vi "Test read multiple pulses.vi"() -> ()   [LabVIEW 2023]
uses:
  <vilib>/DAQmx/create/channels.llb/DAQmx Create Channel (CI-Count Edges).vi
  <vilib>/DAQmx/configure/timing.llb/DAQmx Timing (Sample Clock).vi
  <vilib>/DAQmx/create/channels.llb/DAQmx Create Channel (CO-Pulse Generation-Frequency).vi
  <vilib>/DAQmx/configure/timing.llb/DAQmx Timing (Implicit).vi
  <vilib>/DAQmx/miscellaneous.llb/DAQmx Fill In Error Info.vi
  <vilib>/DAQmx/read.llb/DAQmx Read (Counter 1D U32 1Chan NSamp).vi
  <resource>/objmgr/daqmx.rc
panel:
  out "error out":errorcluster
  in  "# of pulses in train":i32=1000
  out "Actual Duty Cycle":dbl
  out "Actual Frequency":dbl
  in  "Duty Cycle":dbl=0.5 format="%.6f"
  in  "Frequency":dbl=1.0 format="%.6f"
  in  "Output Terminal":tag="/Dev1/PFI12"
  in  "Counter 2":tag="Dev1/ctr0"
  in  "Active Edge":i32(ring)=10280 items=["Rising"=10280, "Falling"=10171]
  in  "Input Terminal":tag="PFI8"
  in  "Counter":tag="Dev1/ctr0"
  in  "Sample Rate":dbl=1000.0
  in  "Sample Clock Source":tag="PFI0"
  in  "Samples per Loop":i32=100
  in  "Stop":bool
  out "Data":u32[](array[numeric])
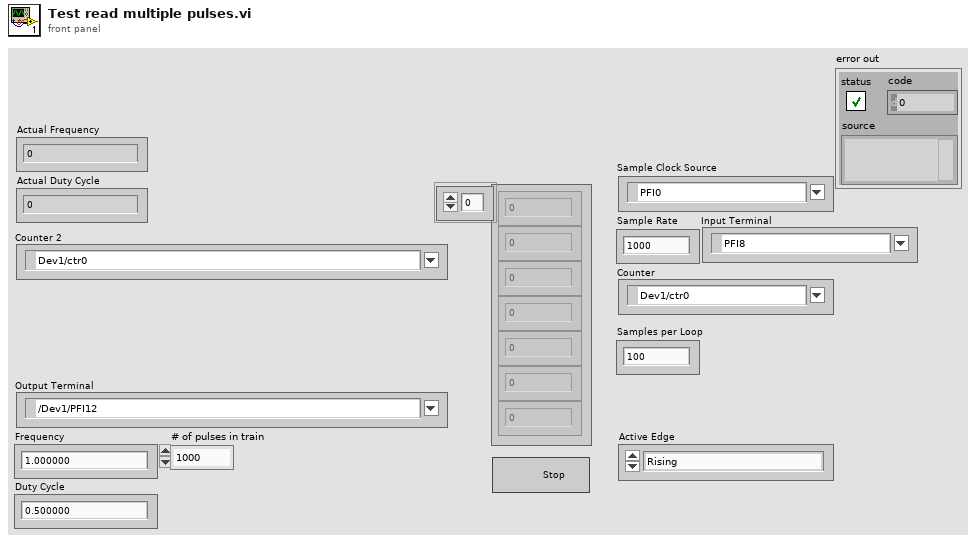
[diagram p1: front panel]
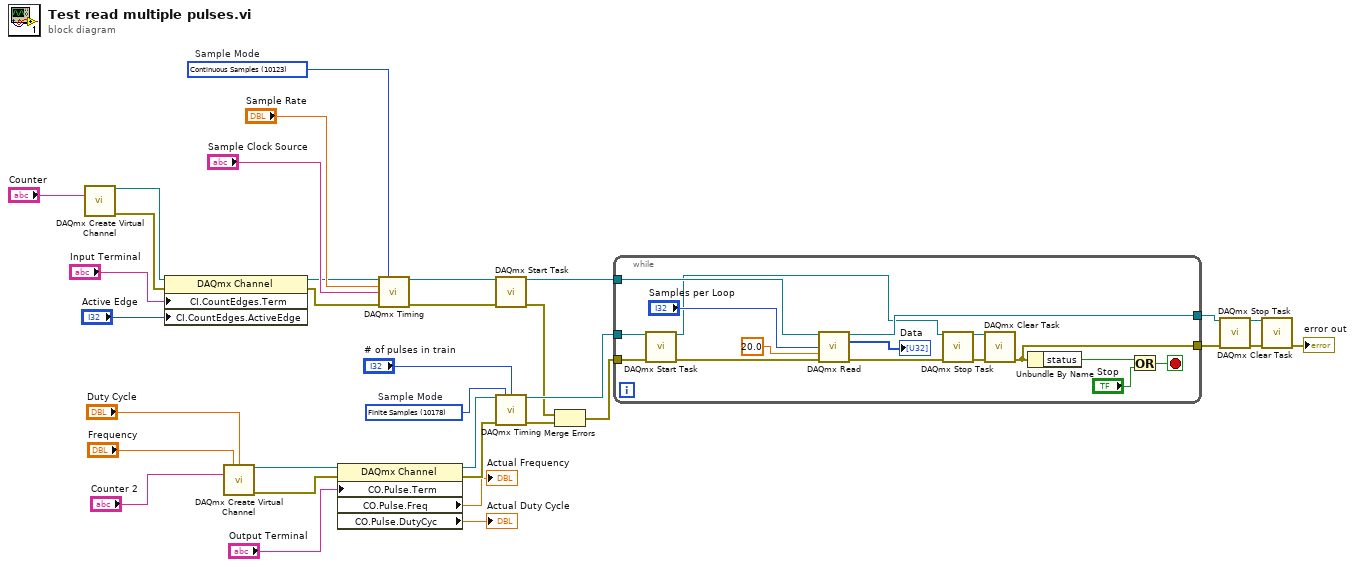
[diagram p0: block diagram]
diagram:
  w17 = 10178 items=["Finite Samples"=10178, "Continuous Samples"=10123, "Hardware Timed Single Point"=12522]  # Sample Mode
  w32 = 10123 items=["Finite Samples"=10178, "Continuous Samples"=10123, "Hardware Timed Single Point"=12522]  # Sample Mode
  n1 = call-poly <vilib>:"DAQmx Create Virtual Channel.vi"("counter"="Counter") -> ("task out"=w27:refnum<k21>, "error out"=w24:errorcluster)  [unwired: 13 in]
  n2 = property class="DAQmx Channel"(reference=w27, error in=w24, "CI.CountEdges.Term"="Input Terminal", "CI.CountEdges.ActiveEdge"="Active Edge") -> (reference out=w26:refnum<k21>, error out=w25:errorcluster)
  n3 = call-poly <vilib>:"DAQmx Create Virtual Channel.vi"("frequency"="Frequency", "duty cycle"="Duty Cycle", "counter"="Counter 2") -> ("task out"=w13:refnum<k21>, "error out"=w12:errorcluster)  [unwired: 11 in]
  n4 = property class="DAQmx Channel"(reference=w13, error in=w12, "CO.Pulse.Term"="Output Terminal") -> (reference out=w9:refnum<k21>, error out=w10:errorcluster, "CO.Pulse.Freq"=→"Actual Frequency":dbl, "CO.Pulse.DutyCyc"=→"Actual Duty Cycle":dbl)
  n5 = call-poly <vilib>:"DAQmx Timing.vi"("task/channels in"=w26, "sample mode"=w32, "rate"="Sample Rate", "source"="Sample Clock Source", "error in"=w25) -> ("task out"=w23:refnum<k21>, "error out"=w22:errorcluster)  [unwired: 9 in]
  n6 = call <vilib>:"DAQmx Start Task.vi"("task/channels in"=w23, "error in"=w22) -> ("task out"=w31:refnum<k21>, "error out"=w2:errorcluster)  [unwired: 12 in]
  n7 = call-poly <vilib>:"DAQmx Timing.vi"("task/channels in"=w9, "sample mode"=w17, "samples per channel"="# of pulses in train", "error in"=w10) -> ("task out"=w15:refnum<k21>, "error out"=w14:errorcluster)  [unwired: 10 in]
  n8 = Merge Errors(w2, w14) -> (w1:errorcluster)
  n9 = while {
    tunnel: w31 -> [w50]
    tunnel: [w36] -> w20
    tunnel: [w48] -> w21
    tunnel: w15 -> [w42]
    tunnel: w1 -> [w35]
    stop <- w49 stop-if-true
    n10 = call <vilib>:"DAQmx Start Task.vi"("task/channels in"=w42, "error in"=w35) -> ("task out"=w37:refnum<k21>, "error out"=w41:errorcluster)  [unwired: 12 in]
    n11 = call-poly <vilib>:"DAQmx Read.vi"("task/channels in"=w50, "number of samples per channel"="Samples per Loop", "timeout"=20.0, "error in"=w41) -> ("task out"=w48:refnum<k21>, "data"=→"Data":u32[], "error out"=w38:errorcluster)  [unwired: 9 in]
    n12 = call <vilib>:"DAQmx Stop Task.vi"("task/channels in"=w37, "error in"=w38) -> ("task out"=w39:refnum<k21>, "error out"=w40:errorcluster)  [unwired: 12 in]
    n13 = call <vilib>:"DAQmx Clear Task.vi"("task in"=w39, "error in"=w40) -> ("error out"=w36:errorcluster)  [unwired: 13 in]
    n14 = Unbundle By Name(w36) -> ("status"=w47:bool)
    n15 = Or(x=w47, y="Stop") -> (x .or. y?=w49:bool)
  }
  n16 = call <vilib>:"DAQmx Stop Task.vi"("task/channels in"=w21, "error in"=w20) -> ("task out"=w18:refnum<k21>, "error out"=w19:errorcluster)  [unwired: 12 in]
  n17 = call <vilib>:"DAQmx Clear Task.vi"("task in"=w18, "error in"=w19) -> ("error out"=→"error out":errorcluster)  [unwired: 13 in]
